vi "FA_ReadETag.vi"(6 "Error In":errorcluster, 8 "ID":string) -> (0 "Error Out":errorcluster, 1 "ETag":string)   [LabVIEW 2014, in "FA_LocalStore.lvlib"]
doc: "Given a Special Type this VI returns that special type's eTag in LocalStore"
uses:
  FA_LocalStore.lvlib
  <vilib>/Utility/config.llb/Read Key (String).vi
  <vilib>/Utility/config.llb/NI_LVConfig.lvlib
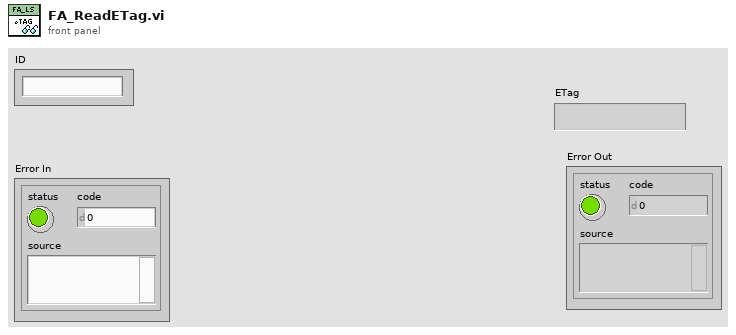
[diagram p1: front panel]
types:
  T1 = typedef "FA_LocalStore.lvlib/FA_LSRef.ctl" = cluster{"eTag INI Refnum":T2, "XML Refnum Array":refnum<file>[]}
  T2 = typedef "NI_LVConfig.lvlib/Config Data RefNum.ctl" = refnum<k1>
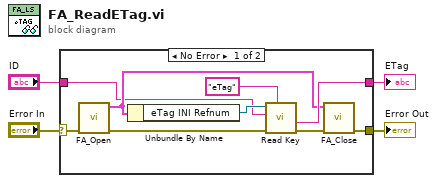
[diagram p0: block diagram]
diagram:
  n1 = case shown="No Error" "Error In" {
    selector: "Error In" -> [w8 w14]
    tunnel: [w9 w14] -> w3
    tunnel: "ID" -> [w6 _]
    tunnel: [w11 _] -> w2
    frame No Error {
      n2 = call "FA_Open.vi"("Error In"=w8) -> ("Error Out"=w5:errorcluster, "FA_LS Ref"=w7:T1)  [unwired: 9 in]
      n3 = Unbundle By Name(w7) -> ("eTag INI Refnum"=w12:T2)
      n4 = call-poly <vilib>:"Read Key.vi"("section"="eTag", "error in (no error)"=w5, "key"=w6, "refnum"=w12) -> ("error out"=w10:errorcluster, "value"=w11:string)  [unwired: 4 in, 2 out]
      n5 = call "FA_Close.vi"("Error In"=w10, "FA_LS Ref"=w7) -> ("Error Out"=w9:errorcluster)  [unwired: 9 in]
    }
    frame Error {
    }
  }
  "Error Out" <- w3
  "ETag" <- w2
